vi "Pulse Mode - Read Duty Cycle.vi"(8 "error in (no error)":errorcluster, 11 "VISA resource name":refnum<visa-resource-name>) -> (0 "error out":errorcluster, 2 "Duty Cycle":u16, 3 "VISA resource name out":refnum<visa-resource-name>)   [LabVIEW 2014, in "Associated Power Technologies 8500 Series.lvlib"]
doc: "Get the setting of duty cycle in pulse mode."
uses:
  <instrlib>/Associated Power Technologies 8500 Series/Associated Power Technologies 8500 Series.lvlib
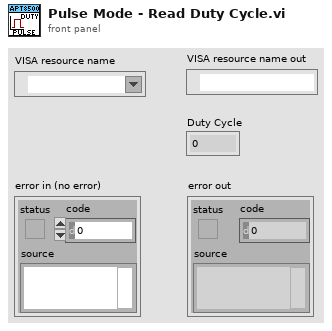
[diagram p1: front panel]
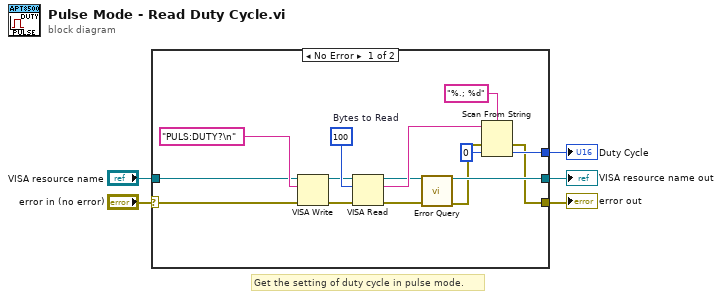
[diagram p0: block diagram]
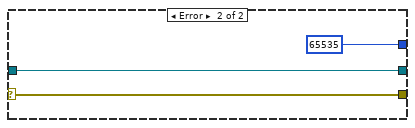
[diagram p2: hidden frame]
diagram:
  # "Get the setting of duty cycle in pulse mode."
  n1 = case shown="No Error" "error in (no error)" {
    selector: "error in (no error)" -> [w16 w23]
    tunnel: [w8 w23] -> w3
    tunnel: [w12 w22] -> w2
    tunnel: "VISA resource name" -> [w15 w22]
    tunnel: [w13 u16 65535] -> w1
    frame No Error {
      w20 = u32 100  # Bytes to Read
      n2 = VISA Write(VISA resource name=w15, write buffer="PULS:DUTY?\n", error in (no error)=w16) -> (VISA resource name out=w18:refnum<visa-resource-name>, error out=w19:errorcluster)  [unwired: 1 out]
      n3 = VISA Read(VISA resource name=w18, byte count=w20, error in (no error)=w19) -> (VISA resource name out=w11:refnum<visa-resource-name>, read buffer=w14:string, error out=w10:errorcluster)  [unwired: 1 out]
      n4 = call <instrlib>:"Error Query.vi"("VISA resource name"=w11, "error in (no error)"=w10) -> ("VISA resource name out"=w12:refnum<visa-resource-name>, "error out"=w9:errorcluster)  [unwired: 10 in, 2 out]
      n5 = Scan From String(format string="%.; %d", input string=w14, error in=w9, default 1=u16 0 ("default value 1")) -> (error out=w8:errorcluster, output 1=w13:u16)  [unwired: 1 in, 2 out]
    }
    frame Error {
    }
  }
  "VISA resource name out" <- w2
  "error out" <- w3
  "Duty Cycle" <- w1
